vi "visa_read.vi"(8 "error in (no error)":errorcluster, 10 "Byte Count (0)":u32, 11 "VISA resource name":refnum<visa-resource-name>) -> (0 "error out":errorcluster, 1 "Data Length":i32, 2 "Read Data":string, 3 "VISA resource name out":refnum<visa-resource-name>)   [LabVIEW 2021, in "Ceyear.lvlib"]
uses:
  <instrlib>/Ceyear/Ceyear.lvlib
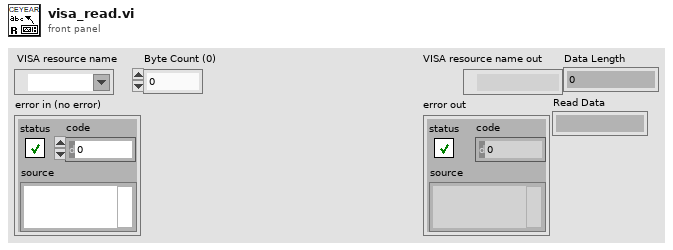
[diagram p1: front panel]
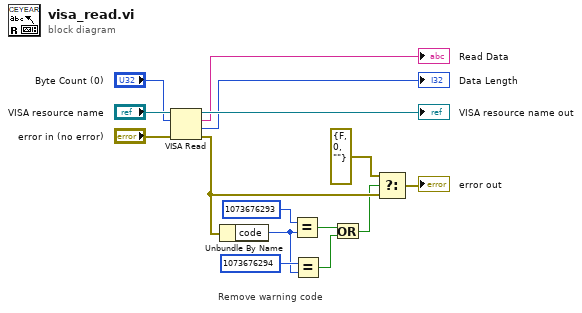
[diagram p0: block diagram]
diagram:
  # "Remove warning code"
  n1 = VISA Read(VISA resource name="VISA resource name", byte count="Byte Count (0)", error in (no error)="error in (no error)") -> (VISA resource name out=→"VISA resource name out":refnum<visa-resource-name>, read buffer=→"Read Data":string, return count=→"Data Length":u32, error out=w10:errorcluster)
  n2 = Unbundle By Name(w10) -> ("code"=w4:i32)
  n3 = Equal?(x=1073676293, y=w4) -> (x = y?=w3:bool)
  n4 = Equal?(x=1073676294, y=w4) -> (x = y?=w2:bool)
  n5 = Or(x=w3, y=w2) -> (x .or. y?=w1:bool)
  n6 = Select(t=errorcluster {"status"=FALSE, "code"=0, "source"=""}, s=w1, f=w10) -> (s? t:f=→"error out":errorcluster)
